vi "ADC Fetch From Digitizing Process.vi"(6 "stop ref":refnum<vi>, 8 "error in":errorcluster, 11 "adc session in":T3={"niScope"={"channel cfg"=[], "sessions"=[], "multi cards"=FALSE, "channels"=0, "type"=enum."n/a", "memory [B/chn]"=0, "ext. clock [Hz]"=0.0, "samples count"=0, "use streaming"=FALSE, "proc setup"={"packet size [smpl]"=0, "current timeout [s]"=0.0, "blk2blk timeout [s]"=0.0, "event time"=timestamp(0 s since 1904-01-01), "temp sampl T [s]"=0.0, "data queue"=refnum, "stop notifier"=refnum, "proc ref"=refnum}, "sample width [B]"=0, "ranges [V]"=[], "trigger setup"={"coupling"=1, "level [V]"=0.0, "slope"=0, "mode"=enum."Immediate"}, "fs [Hz]"=0.0, "bitres [bit]"=0}, "3458A"={"channels"=[], "sync unit"={"VISA"="", "type"=enum."Picotest U6200A"}, "awg unit"={"type"=enum."Agilent 331xxA to 332xxA", "VISA"="", "enable 10MHz ref"=FALSE}, "sync mode"=enum."MASTER-SLAVE, MASTER clocked by TIMER", "streaming mode"=FALSE, "idn mode"=enum."Auto", "sampling mode"=enum."DCV", "Ts [s]"=0.0, "sample memory [B]"=0, "proc setup"={"channel id"=0, "packet size [smpl]"=0, "current timeout [s]"=0.0, "blk2blk timeout [s]"=0.0, "event time"=timestamp(0 s since 1904-01-01), "stop notifier"=refnum, "data queues"=[], "proc refs"=[], "bus semaphore"=refnum}, "sample size [B]"=0, "sample count"=0, "aux data"={"channel id"=0, "valid?"=[], "gain [V]"=[], "timestamp [s]"=[], "Ts [s]"=0.0, "abs timestamp"=timestamp(0 s since 1904-01-01), "t [deg C]"=[]}, "ranges [V]"=[], "aperture [s]"=0.0, "LEVEL trigger"={"edge"=enum."POS", "level [V]"=0.0, "coupling"=enum."DC"}, "trigger mode"=enum."AUTO", "measure temp.?"=FALSE, "disp mesages"=[], "shared bus?"=FALSE, "disable display?"=FALSE, "aper mode"=enum."Manual", "aper rules"=[]}, "dsdll"={"dsdll"={"dsdll path"=path "", "dsdll handle"=[], "output devices"=[], "capture devices"=[]}, "channels"=0, "device id"=0, "channel idns"=[], "proc setup"={"packet size [smpl]"=0, "current timeout [s]"=0.0, "blk2blk timeout [s]"=0.0, "event time"=timestamp(0 s since 1904-01-01), "data queue"=refnum, "stop notifier"=refnum, "proc ref"=refnum}, "samples count"=0, "fs [Hz]"=0.0}, "type"=enum."niScope", "channel idn str"=[], "aux instr idn str"=[], "modified?"=FALSE, "simadc"={"channels"=[], "range [V]"=0.0, "Ts step [s]"=0.0, "time [s]"=0.0, "fs [Hz]"=0.0, "count"=0, "smpl offset"=0, "set count"=0, "bit res"=0}, "force rst?"=FALSE, "exit mode"=enum."Immediate reset", "exit dly"=0.0, "exit tmr"=timestamp(0 s since 1904-01-01), "busy?"=FALSE, "accessed?"=FALSE, "QuADC session"={"channel cfg"=[], "sessions"=[], "multi cards"=FALSE, "channels"=0, "type"=enum."n/a", "memory [B/chn]"=0, "ext. clock [Hz]"=0.0, "samples count"=0, "use streaming"=FALSE, "proc setup"={"packet size [smpl]"=0, "current timeout [s]"=0.0, "blk2blk timeout [s]"=0.0, "event time"=timestamp(0 s since 1904-01-01), "temp sampl T [s]"=0.0, "data queue"=refnum, "stop notifier"=refnum, "proc ref"=refnum}, "sample width [B]"=0, "ranges [V]"=[], "trigger setup"={"coupling"=1, "level [V]"=0.0, "slope"=0, "mode"=enum."Immediate"}, "fs [Hz]"=0.0, "bitres [bit]"=0}} {"QuADC session"."trigger setup"."level [V]" format="%.2f"; "QuADC session"."trigger setup"."coupling" items=["AC"=0, "DC"=1, "HF Reject"=3, "LF Reject"=4, "AC Plus HF Reject"=1001]; "QuADC session"."channel cfg"."Clock fr. (Hz)" min=0.0 format="%#_9p"; "QuADC session"."channel cfg"."Number of JJ" min=1; "QuADC session"."channel cfg"."Range [Vpk]" min=0.0; "QuADC session"."channel cfg"."Channel" min=0; "3458A"."channels"."Range [Vpk]" min=0.0; "niScope"."trigger setup"."level [V]" format="%.2f"; "niScope"."trigger setup"."coupling" items=["AC"=0, "DC"=1, "HF Reject"=3, "LF Reject"=4, "AC Plus HF Reject"=1001]; "niScope"."channel cfg"."Range [Vpk]" min=0.0; "niScope"."channel cfg"."Channel" min=0}) -> (0 "error out":errorcluster, 1 "aux data":T1, 2 "data packet":T2, 3 "adc session out":T3={"niScope"={"channel cfg"=[], "sessions"=[], "multi cards"=FALSE, "channels"=0, "type"=enum."n/a", "memory [B/chn]"=0, "ext. clock [Hz]"=0.0, "samples count"=0, "use streaming"=FALSE, "proc setup"={"packet size [smpl]"=0, "current timeout [s]"=0.0, "blk2blk timeout [s]"=0.0, "event time"=timestamp(0 s since 1904-01-01), "temp sampl T [s]"=0.0, "data queue"=refnum, "stop notifier"=refnum, "proc ref"=refnum}, "sample width [B]"=0, "ranges [V]"=[], "trigger setup"={"coupling"=1, "level [V]"=0.0, "slope"=0, "mode"=enum."Immediate"}, "fs [Hz]"=0.0, "bitres [bit]"=0}, "3458A"={"channels"=[], "sync unit"={"VISA"="", "type"=enum."Picotest U6200A"}, "awg unit"={"type"=enum."Agilent 331xxA to 332xxA", "VISA"="", "enable 10MHz ref"=FALSE}, "sync mode"=enum."MASTER-SLAVE, MASTER clocked by TIMER", "streaming mode"=FALSE, "idn mode"=enum."Auto", "sampling mode"=enum."DCV", "Ts [s]"=0.0, "sample memory [B]"=0, "proc setup"={"channel id"=0, "packet size [smpl]"=0, "current timeout [s]"=0.0, "blk2blk timeout [s]"=0.0, "event time"=timestamp(0 s since 1904-01-01), "stop notifier"=refnum, "data queues"=[], "proc refs"=[], "bus semaphore"=refnum}, "sample size [B]"=0, "sample count"=0, "aux data"={"channel id"=0, "valid?"=[], "gain [V]"=[], "timestamp [s]"=[], "Ts [s]"=0.0, "abs timestamp"=timestamp(0 s since 1904-01-01), "t [deg C]"=[]}, "ranges [V]"=[], "aperture [s]"=0.0, "LEVEL trigger"={"edge"=enum."POS", "level [V]"=0.0, "coupling"=enum."DC"}, "trigger mode"=enum."AUTO", "measure temp.?"=FALSE, "disp mesages"=[], "shared bus?"=FALSE, "disable display?"=FALSE, "aper mode"=enum."Manual", "aper rules"=[]}, "dsdll"={"dsdll"={"dsdll path"=path "", "dsdll handle"=[], "output devices"=[], "capture devices"=[]}, "channels"=0, "device id"=0, "channel idns"=[], "proc setup"={"packet size [smpl]"=0, "current timeout [s]"=0.0, "blk2blk timeout [s]"=0.0, "event time"=timestamp(0 s since 1904-01-01), "data queue"=refnum, "stop notifier"=refnum, "proc ref"=refnum}, "samples count"=0, "fs [Hz]"=0.0}, "type"=enum."niScope", "channel idn str"=[], "aux instr idn str"=[], "modified?"=FALSE, "simadc"={"channels"=[], "range [V]"=0.0, "Ts step [s]"=0.0, "time [s]"=0.0, "fs [Hz]"=0.0, "count"=0, "smpl offset"=0, "set count"=0, "bit res"=0}, "force rst?"=FALSE, "exit mode"=enum."Immediate reset", "exit dly"=0.0, "exit tmr"=timestamp(0 s since 1904-01-01), "busy?"=FALSE, "accessed?"=FALSE, "QuADC session"={"channel cfg"=[], "sessions"=[], "multi cards"=FALSE, "channels"=0, "type"=enum."n/a", "memory [B/chn]"=0, "ext. clock [Hz]"=0.0, "samples count"=0, "use streaming"=FALSE, "proc setup"={"packet size [smpl]"=0, "current timeout [s]"=0.0, "blk2blk timeout [s]"=0.0, "event time"=timestamp(0 s since 1904-01-01), "temp sampl T [s]"=0.0, "data queue"=refnum, "stop notifier"=refnum, "proc ref"=refnum}, "sample width [B]"=0, "ranges [V]"=[], "trigger setup"={"coupling"=1, "level [V]"=0.0, "slope"=0, "mode"=enum."Immediate"}, "fs [Hz]"=0.0, "bitres [bit]"=0}} {"QuADC session"."trigger setup"."level [V]" format="%.2f"; "QuADC session"."trigger setup"."coupling" items=["AC"=0, "DC"=1, "HF Reject"=3, "LF Reject"=4, "AC Plus HF Reject"=1001]; "QuADC session"."channel cfg"."Clock fr. (Hz)" min=0.0 format="%#_9p"; "QuADC session"."channel cfg"."Number of JJ" min=1; "QuADC session"."channel cfg"."Range [Vpk]" min=0.0; "QuADC session"."channel cfg"."Channel" min=0; "3458A"."channels"."Range [Vpk]" min=0.0; "niScope"."trigger setup"."level [V]" format="%.2f"; "niScope"."trigger setup"."coupling" items=["AC"=0, "DC"=1, "HF Reject"=3, "LF Reject"=4, "AC Plus HF Reject"=1001]; "niScope"."channel cfg"."Range [Vpk]" min=0.0; "niScope"."channel cfg"."Channel" min=0}, 4 "fetching done?":bool)   [LabVIEW 2018]
doc: "Call this in a loop to fetch sample data comming from running digitizing process(es). It fetches the sample data, merges them from particular channels to one array.\nIf some sample data are available or a status is updated it will be found in 'data packet' variable. Content of the variable is valid only if its flag 'valid?' is true. It contains data either in int32 or int16 format. Everytime some data are returned the 'count' of samples per channels is non-zero and 'offset' indicates relative position of first sample to the start of sampling. When digitizer is sampling (not just returning data) the flag 'sampling' is true. If supported by selected HW it will also return usage of intrument memory buffer and sample data queue. If not supported the value will be NaN. \nSecond output of the VI is 'aux data' which are returned only once per whole fetching sequence. It is valid if its flag 'valid?' is True. The aux. data contains 'gain' and 'offset' scaling factors needed to convert integer sample data to voltage. It will also return vector of measured temperatures and corresponding timestamps of measurement during the sampling if it is supported by the HW. Last parameter is a relative timestamp of first sample for each channel. \nCaller must check and process content of both 'data packet' and 'aux data' every time this VI is called. Fetching must be terminated when the function returnes error or returnes True on 'fetching done?' flag.\nVI modifies session content so do not assign just ADC session in!"
uses:
  ADC Session.ctl
  drivers/niScope/niScope Session.ctl
  drivers/niScope/niScope Virtual Channel Config.ctl
  drivers/niScope/niScope Virtual Channel Mode.ctl
  drivers/niScope/niScope Virtual Channel Input Z.ctl
  drivers/niScope/niScope Virtual Channel Coupling.ctl
  drivers/niScope/niScope Type.ctl
  drivers/niScope/niScope Digitizing Process Options.ctl
  drivers/niScope/niScope Data Packet.ctl
  drivers/niScope/niScope Trigger Setup.ctl
  <instrlib>/niScope/Controls/niScope trigger coupling.ctl
  <instrlib>/niScope/Controls/niScope trigger slope.ctl
  drivers/DMM/3458A Digitizer Session.ctl
  drivers/DMM/3458A Virtual Channel Config.ctl
  drivers/Counter/Counter Session.ctl
  drivers/Counter/Counter Type.ctl
  drivers/AWG/AWG Session.ctl
  drivers/AWG/AWG Type.ctl
  drivers/DMM/3458A Sync Mode.ctl
  drivers/DMM/3458A Idn Mode.ctl
  drivers/DMM/3458A Digitizing Low Levels/Configure/Sampling Mode.ctl
  drivers/DMM/3458A Digitizing Process Options.ctl
  drivers/DMM/3458A Data Packet.ctl
  drivers/DMM/3458A Aux Record Data.ctl
  drivers/DMM/3458A Digitizing Low Levels/Configure/Level Setup.ctl
  drivers/DMM/3458A Digitizing Low Levels/Configure/First Sample Trigger.ctl
  drivers/DMM/3458A Aperture Selection Mode.ctl
  drivers/dsdll/DSDLL Session.ctl
  drivers/dsdll/dsdll source distribution/dsdll_instance.ctl
  drivers/dsdll/dsdll source distribution/dsdll_device_record.ctl
  drivers/dsdll/DSDLL Process Config.ctl
  drivers/dsdll/DSDLL Data Packet.ctl
  ADC Type.ctl
  drivers/simulated_adc/SimAdc Config.ctl
  drivers/simulated_adc/SimAdc Channel Cfg.ctl
  ADC On Close Action.ctl
  drivers/Quatsch_driver/QuADCDriver/QuADC Session.ctl
  drivers/Quatsch_driver/QuADCDriver/QuADC Virtual Channel Config.ctl
  drivers/Quatsch_driver/QuADCDriver/QuADC Virtual Channel Mode.ctl
  drivers/Quatsch_driver/QuADCDriver/QuADC Virtual Channel Input Z.ctl
  drivers/Quatsch_driver/QuADCDriver/QuADC Virtual Channel Coupling.ctl
  drivers/Quatsch_driver/QuADCDriver/QuADC Type.ctl
  drivers/Quatsch_driver/QuADCDriver/QuADC Digitizing Process Options.ctl
  drivers/Quatsch_driver/QuADCDriver/QuADC Data Packet.ctl
  drivers/Quatsch_driver/QuADCDriver/QuADC Trigger Setup.ctl
  ADC Data Packet.ctl
  ADC Aux Data.ctl
  drivers/niScope/niScope Virtual Digitizer.lvlib
  drivers/DMM/3458A Virtual Digitizer.lvlib
  drivers/dsdll/DSDLL Virtual Digitizer.lvlib
  <vilib>/Utility/error.llb/Error Cluster From Error Code.vi
  <vilib>/ErrorRing/Error Ring.xnode
  drivers/Quatsch_driver/QuADCDriver/QuADC Virtual Digitizer.lvlib
  drivers/Counter/Counter.lvlib
  drivers/AWG/AWG.lvlib
  drivers/DMM/3458A Digitizing Low Levels/3458A Digitizing Low Levels.lvlib
  drivers/dsdll/dsdll source distribution/dsdll.lvlib
panel:
  # "IP Address"
  # "."
  # "."
  # "."
  # ":"
  # "IP Address"
  # "."
  # "."
  # "."
  # ":"
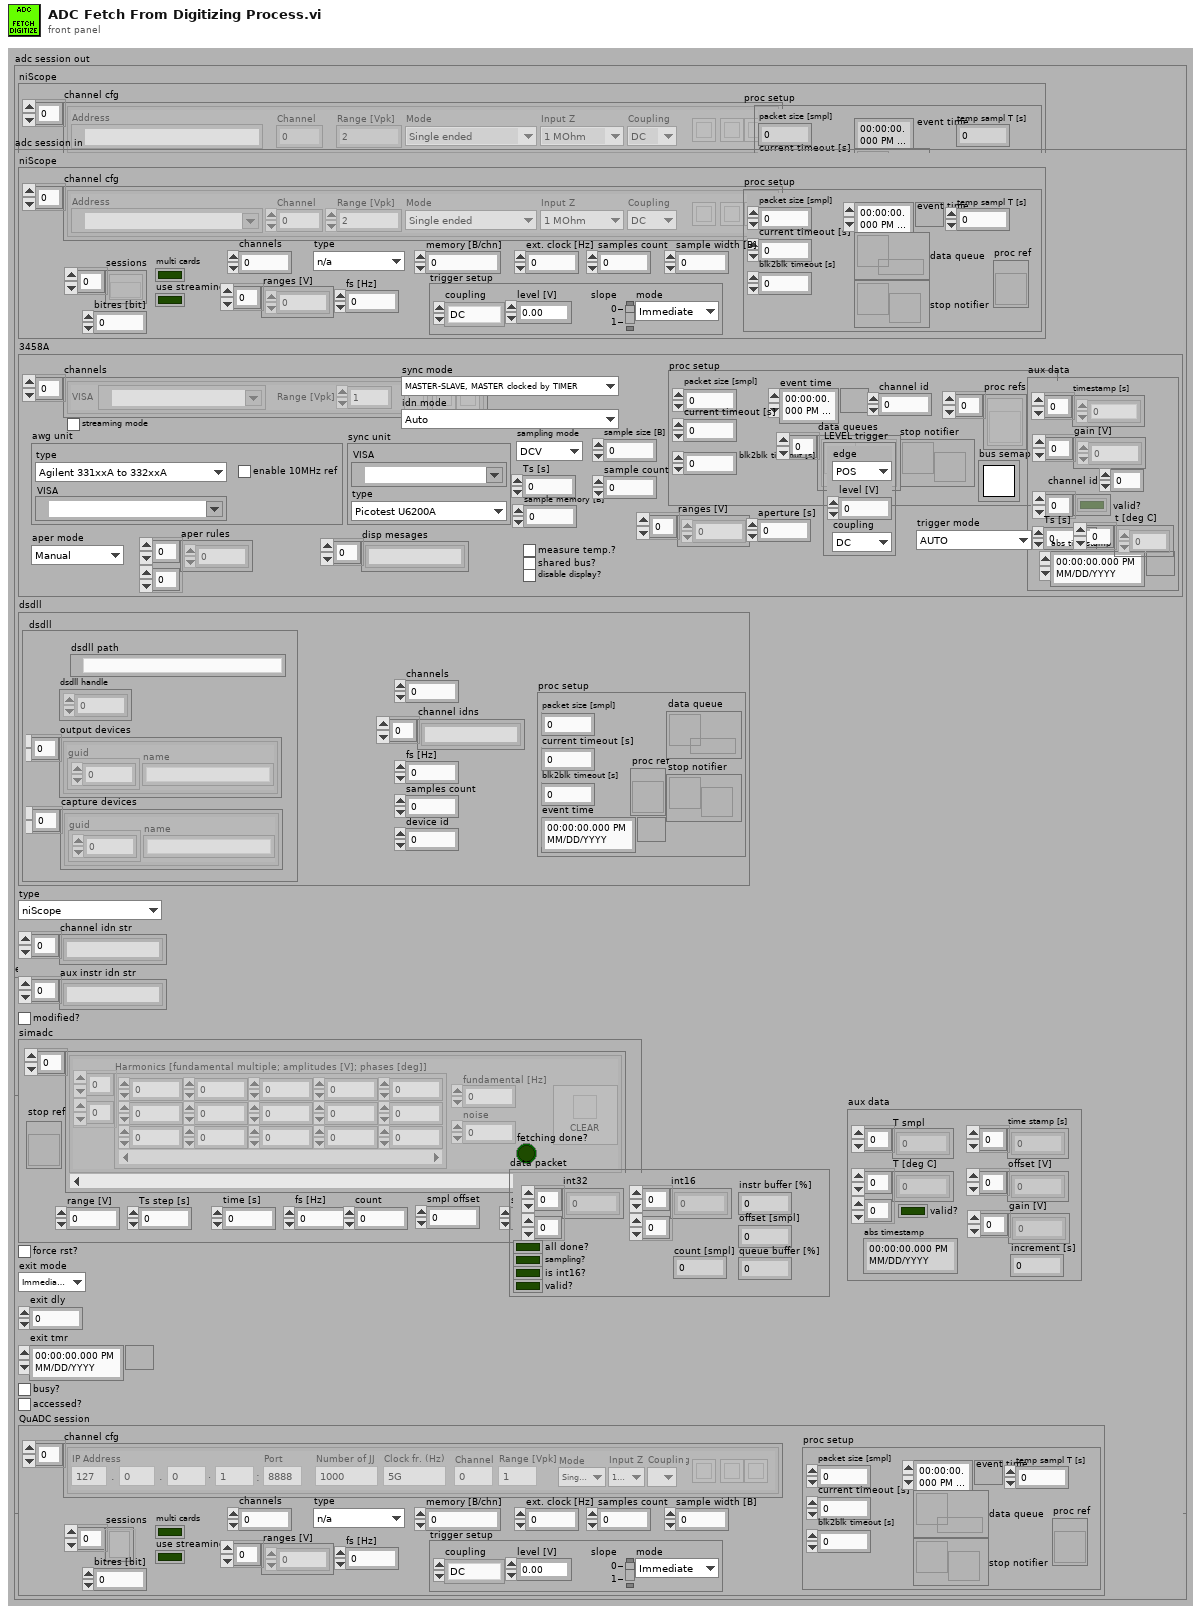
[diagram p1: front panel]
types:
  T1 = typedef "ADC Aux Data.ctl" = cluster{"offset [V]":dbl[], "gain [V]":dbl[], "time stamp [s]":dbl[], "increment [s]":dbl, "T smpl":i64[], "T [deg C]":dbl[][], "valid?":bool, "abs timestamp":timestamp}
  T2 = typedef "ADC Data Packet.ctl" = cluster{"int32":i32[][], "int16":i16[][], "offset [smpl]":i64, "count [smpl]":i32, "is int16?":bool, "all done?":bool, "sampling?":bool, "instr buffer [%]":dbl, "queue buffer [%]":dbl, "valid?":bool}
  T3 = typedef "ADC Session.ctl" = cluster{"niScope":T4, "3458A":T14, "dsdll":T29, "type":T33, "channel idn str":string[], "aux instr idn str":string[], "modified?":bool, "simadc":T34, "force rst?":bool, "exit mode":T36, "exit dly":dbl, "exit tmr":timestamp, "busy?":bool, "accessed?":bool, "QuADC session":T37}
  T4 = typedef "niScope Virtual Digitizer.lvlib/niScope Session.ctl" = cluster{"channel cfg":T5[], "sessions":refnum<k20>[], "multi cards":bool, "channels":i32, "type":T9, "memory [B/chn]":i32, "ext. clock [Hz]":dbl, "samples count":i64, "use streaming":bool, "proc setup":T10, "sample width [B]":i32, "ranges [V]":dbl[], "trigger setup":T11, "fs [Hz]":dbl, "bitres [bit]":i32}
  T5 = typedef "niScope Virtual Digitizer.lvlib/niScope Virtual Channel Config.ctl" = cluster{"Address":refnum<k15>, "Channel":i32, "Mode":T6, "Input Z":T7, "Coupling":T8, "Range [Vpk]":dbl, "btn clr":bool, "btn up":bool, "btn down":bool}
  T6 = typedef "niScope Virtual Digitizer.lvlib/niScope Virtual Channel Mode.ctl" = enum16{"Single ended", "Unbal. differential", "Differential"}
  T7 = typedef "niScope Virtual Digitizer.lvlib/niScope Virtual Channel Input Z.ctl" = enum16{"1 MOhm", "50 Ohm"}
  T8 = typedef "niScope Virtual Digitizer.lvlib/niScope Virtual Channel Coupling.ctl" = enum16{"AC", "DC", "GND"}
  T9 = typedef "niScope Virtual Digitizer.lvlib/niScope Type.ctl" = enum16{"n/a", "5922"}
  T10 = typedef "niScope Virtual Digitizer.lvlib/niScope Digitizing Process Options.ctl" = cluster{"packet size [smpl]":i64, "current timeout [s]":dbl, "blk2blk timeout [s]":dbl, "event time":timestamp, "temp sampl T [s]":dbl, "data queue":refnum<queue>, "stop notifier":refnum<notifier>, "proc ref":refnum<vi>}
  T11 = typedef "niScope Virtual Digitizer.lvlib/niScope Trigger Setup.ctl" = cluster{"coupling":T12, "level [V]":dbl, "slope":T13, "mode":enum16{"Immediate", "External", "Level"}}
  T12 = typedef "niScope trigger coupling.ctl" = u16
  T13 = typedef "niScope trigger slope.ctl" = i32
  T14 = typedef "3458A Virtual Digitizer.lvlib/3458A Digitizer Session.ctl" = cluster{"channels":T15[], "sync unit":T16, "awg unit":T18, "sync mode":T20, "streaming mode":bool, "idn mode":T21, "sampling mode":T22, "Ts [s]":dbl, "sample memory [B]":i32, "proc setup":T23, "sample size [B]":i32, "sample count":i32, "aux data":T25, "ranges [V]":dbl[], "aperture [s]":dbl, "LEVEL trigger":T26, "trigger mode":T27, "measure temp.?":bool, "disp mesages":string[], "shared bus?":bool, "disable display?":bool, "aper mode":T28, "aper rules":dbl[][]}
  T15 = typedef "3458A Virtual Digitizer.lvlib/3458A Virtual Channel Config.ctl" = cluster{"VISA":refnum<visa-resource-name>, "Range [Vpk]":dbl, "btn clr":bool, "btn up":bool, "btn down":bool}
  T16 = typedef "Counter.lvlib/Counter Session.ctl" = cluster{"VISA":refnum<visa-resource-name>, "type":T17}
  T17 = typedef "Counter.lvlib/Counter Type.ctl" = enum16{"Picotest U6200A", "dummy"}
  T18 = typedef "AWG.lvlib/AWG Session.ctl" = cluster{"type":T19, "VISA":refnum<visa-resource-name>, "enable 10MHz ref":bool}
  T19 = typedef "AWG.lvlib/AWG Type.ctl" = enum16{"Agilent 331xxA to 332xxA", "Agilent 335xxA to 336xxA", "Tektronix AFG3101C", "dummy"}
  T20 = typedef "3458A Virtual Digitizer.lvlib/3458A Sync Mode.ctl" = enum16{"MASTER-SLAVE, MASTER clocked by TIMER", "MASTER-SLAVE, MASTER clocked by AWG", "ALL clocked by AWG", "MASTER-SLAVE, ALL clocked by TIMER", "ALL clocked by AWG with DFLL"}
  T21 = typedef "3458A Virtual Digitizer.lvlib/3458A Idn Mode.ctl" = enum16{"Auto", "Sequential (chn A, chn B, ...)", "From calibration string"}
  T22 = typedef "3458A Virtual Digitizer.lvlib/3458A Digitizing Low Levels.lvlib/Sampling Mode.ctl" = enum16{"DCV", "DSDC", "DSAC"}
  T23 = typedef "3458A Virtual Digitizer.lvlib/3458A Digitizing Process Options.ctl" = cluster{"channel id":i32, "packet size [smpl]":i32, "current timeout [s]":dbl, "blk2blk timeout [s]":dbl, "event time":timestamp, "stop notifier":refnum<notifier>, "data queues":refnum<queue>[], "proc refs":refnum<vi>[], "bus semaphore":T24}
  T24 = typedef "Semaphore RefNum" = refnum<k1>
  T25 = typedef "3458A Virtual Digitizer.lvlib/3458A Aux Record Data.ctl" = cluster{"channel id":i32, "valid?":bool[], "gain [V]":dbl[], "timestamp [s]":dbl[], "Ts [s]":dbl, "abs timestamp":timestamp, "t [deg C]":dbl[]}
  T26 = typedef "3458A Virtual Digitizer.lvlib/3458A Digitizing Low Levels.lvlib/Level Setup.ctl" = cluster{"edge":enum16{"POS", "NEG"}, "level [V]":dbl, "coupling":enum16{"DC", "AC"}}
  T27 = typedef "3458A Virtual Digitizer.lvlib/3458A Digitizing Low Levels.lvlib/First Sample Trigger.ctl" = enum16{"AUTO", "EXT", "SYN", "SGL", "HOLD", "LEVEL"}
  T28 = typedef "3458A Virtual Digitizer.lvlib/3458A Aperture Selection Mode.ctl" = enum16{"Manual", "Maximum", "Table"}
  T29 = typedef "DSDLL Virtual Digitizer.lvlib/DSDLL Session.ctl" = cluster{"dsdll":T30, "channels":i32, "device id":i32, "channel idns":string[], "proc setup":T32, "samples count":i32, "fs [Hz]":dbl}
  T30 = typedef "dsdll.lvlib/dsdll_instance.ctl" = cluster{"dsdll path":path, "dsdll handle":u8[], "output devices":T31[], "capture devices":T31[]}
  T31 = typedef "dsdll.lvlib/dsdll_device_record.ctl" = cluster{"guid":u8[], "name":string}
  T32 = typedef "DSDLL Virtual Digitizer.lvlib/DSDLL Process Config.ctl" = cluster{"packet size [smpl]":i32, "current timeout [s]":dbl, "blk2blk timeout [s]":dbl, "event time":timestamp, "data queue":refnum<queue>, "stop notifier":refnum<notifier>, "proc ref":refnum<vi>}
  T33 = typedef "ADC Type.ctl" = enum16{"niScope", "3458A", "DirectSound DLL", "dummy", "QuADC"}
  T34 = typedef "SimAdc Config.ctl" = cluster{"channels":T35[], "range [V]":dbl, "Ts step [s]":dbl, "time [s]":dbl, "fs [Hz]":dbl, "count":i64, "smpl offset":i64, "set count":i64, "bit res":i32}
  T35 = typedef "SimAdc Channel Cfg.ctl" = cluster{"harmonics":dbl[][], "btn clear":bool, "noise":dbl, "fundamental [Hz]":dbl}
  T36 = typedef "ADC On Close Action.ctl" = enum16{"Immediate reset", "Delayed reset"}
  T37 = typedef "QuADC Virtual Digitizer.lvlib/QuADC Session.ctl" = cluster{"channel cfg":T38[], "sessions":refnum<k5>[], "multi cards":bool, "channels":i32, "type":T42, "memory [B/chn]":i32, "ext. clock [Hz]":dbl, "samples count":i64, "use streaming":bool, "proc setup":T43, "sample width [B]":i32, "ranges [V]":dbl[], "trigger setup":T44, "fs [Hz]":dbl, "bitres [bit]":i32}
  T38 = typedef "QuADC Virtual Digitizer.lvlib/QuADC Virtual Channel Config.ctl" = cluster{"Channel":i32, "Mode":T39, "Input Z":T40, "Coupling":T41, "Range [Vpk]":dbl, "btn clr":bool, "btn up":bool, "btn down":bool, "IP address A":u8, "IP address B":u8, "IP address C":u8, "IP address D":u8, "Port":u16, "Number of JJ":u32, "Clock fr. (Hz)":dbl}
  T39 = typedef "QuADC Virtual Digitizer.lvlib/QuADC Virtual Channel Mode.ctl" = enum16{"Single ended", "Unbal. differential", "Differential"}
  T40 = typedef "QuADC Virtual Digitizer.lvlib/QuADC Virtual Channel Input Z.ctl" = enum16{"1 MOhm", "50 Ohm"}
  T41 = typedef "QuADC Virtual Digitizer.lvlib/QuADC Virtual Channel Coupling.ctl" = enum16{"AC", "DC", "GND"}
  T42 = typedef "QuADC Virtual Digitizer.lvlib/QuADC Type.ctl" = enum16{"n/a", "v1"}
  T43 = typedef "QuADC Virtual Digitizer.lvlib/QuADC Digitizing Process Options.ctl" = cluster{"packet size [smpl]":i64, "current timeout [s]":dbl, "blk2blk timeout [s]":dbl, "event time":timestamp, "temp sampl T [s]":dbl, "data queue":refnum<queue>, "stop notifier":refnum<notifier>, "proc ref":refnum<vi>}
  T44 = typedef "QuADC Virtual Digitizer.lvlib/QuADC Trigger Setup.ctl" = cluster{"coupling":T12, "level [V]":dbl, "slope":T13, "mode":enum16{"Immediate", "External", "Level"}}
  T45 = typedef "niScope Virtual Digitizer.lvlib/niScope Record Aux Data.ctl" = cluster{"T smpl":i64[], "T [deg C]":dbl[][], "time stamp [s]":dbl[], "offset":dbl[], "gain":dbl[], "increment [s]":dbl, "valid?":bool, "abs timestamp":timestamp}
  T46 = typedef "niScope Virtual Digitizer.lvlib/niScope Data Packet.ctl" = cluster{"int32":i32[][], "card buffer [%]":dbl, "all done?":bool, "offset [smpl]":i64, "sampling?":bool, "queue buffer [%]":dbl, "int16":i16[][], "is int16?":bool, "count [smpl]":i32, "valid?":bool}
  T47 = typedef "QuADC Virtual Digitizer.lvlib/QuADC Record Aux Data.ctl" = cluster{"T smpl":i64[], "T [deg C]":dbl[][], "time stamp [s]":dbl[], "offset":dbl[], "gain":dbl[], "increment [s]":dbl, "valid?":bool, "abs timestamp":timestamp}
  T48 = typedef "QuADC Virtual Digitizer.lvlib/QuADC Data Packet.ctl" = cluster{"int32":i32[][], "card buffer [%]":dbl, "all done?":bool, "offset [smpl]":i64, "sampling?":bool, "queue buffer [%]":dbl, "int16":i16[][], "is int16?":bool, "count [smpl]":i32, "valid?":bool}
  T49 = typedef "3458A Virtual Digitizer.lvlib/3458A Data Packet.ctl" = cluster{"data":i32[][], "offset [smpl]":i32, "count [smpl]":i32, "all done?":bool, "sampling?":bool, "queue buffer [%]":dbl, "valid?":bool}
  T50 = typedef "DSDLL Virtual Digitizer.lvlib/DSDLL Aux Record Data.ctl" = cluster{"time stamp [s]":dbl[], "gain":dbl[], "increment [s]":dbl, "valid?":bool, "abs timestamp":timestamp}
  T51 = typedef "DSDLL Virtual Digitizer.lvlib/DSDLL Data Packet.ctl" = cluster{"int32":i32[][], "card buffer [%]":dbl, "all done?":bool, "offset [smpl]":i32, "sampling?":bool, "queue buffer [%]":dbl, "count [smpl]":i32, "valid?":bool}
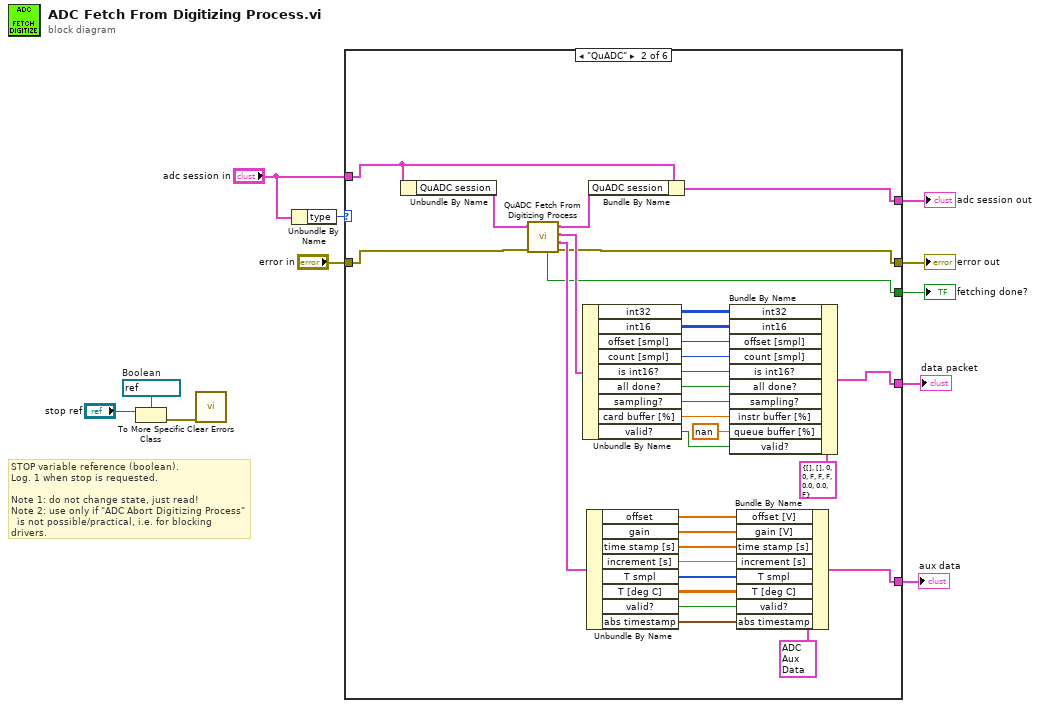
[diagram p0: block diagram]
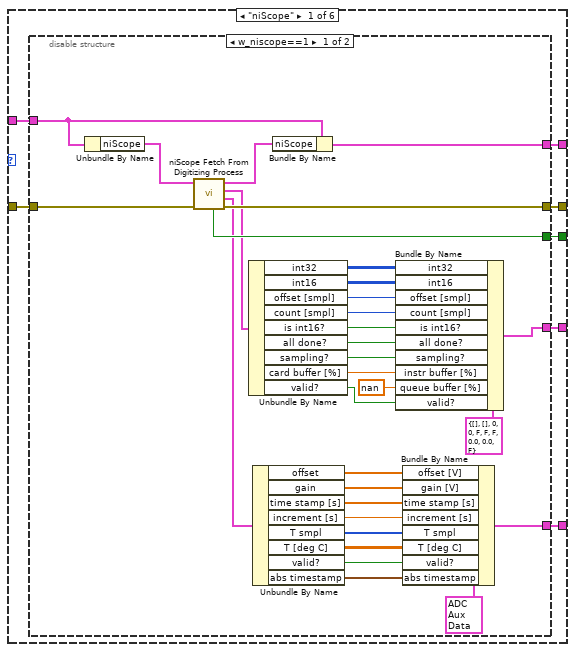
[diagram p2: hidden frame]
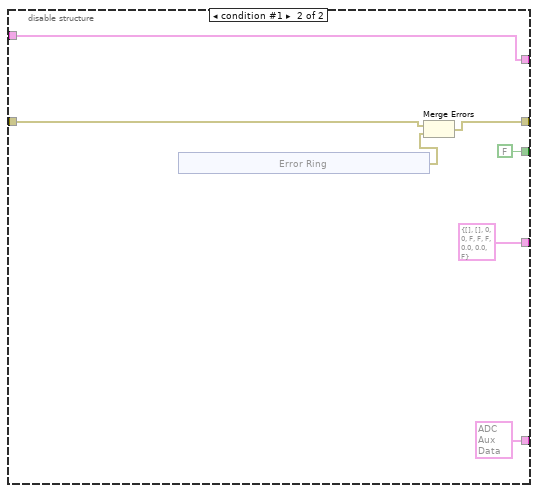
[diagram p3: hidden frame]
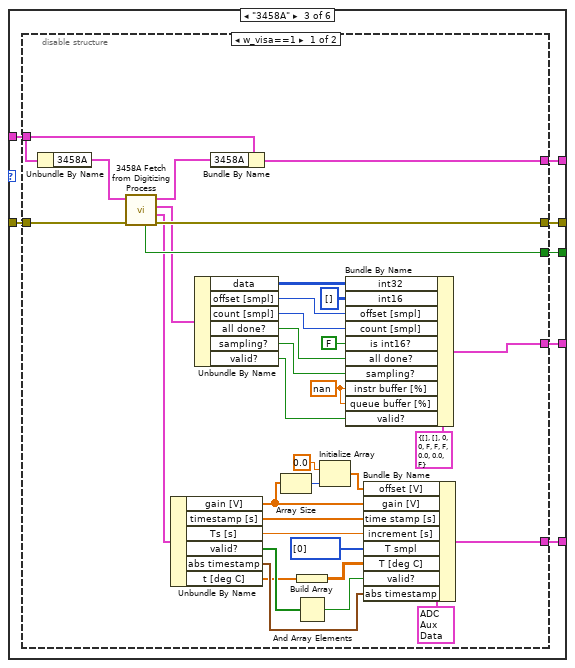
[diagram p4: hidden frame]
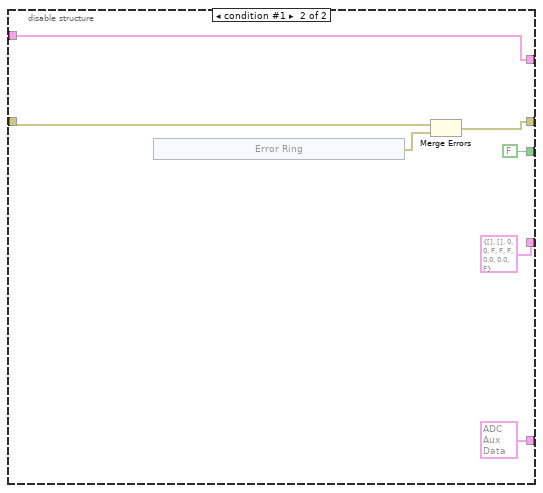
[diagram p5: hidden frame]
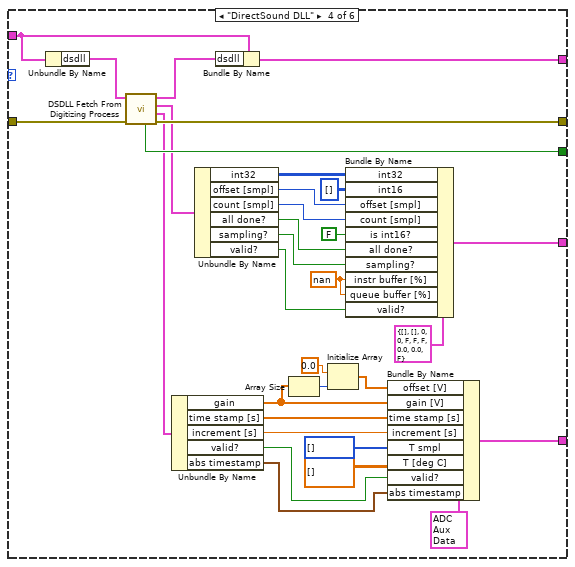
[diagram p6: hidden frame]
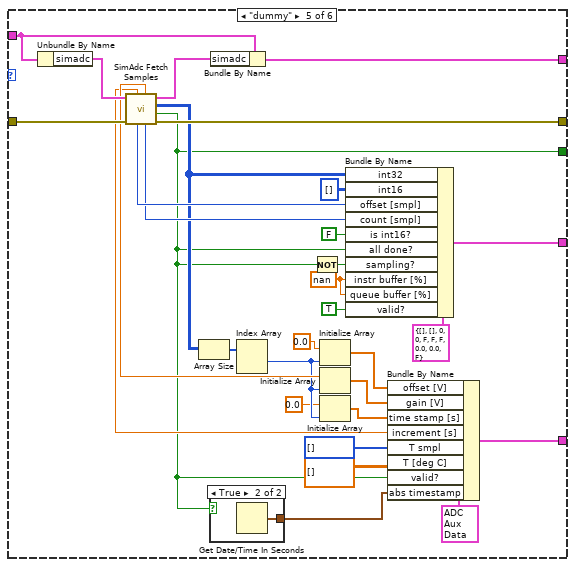
[diagram p7: hidden frame]
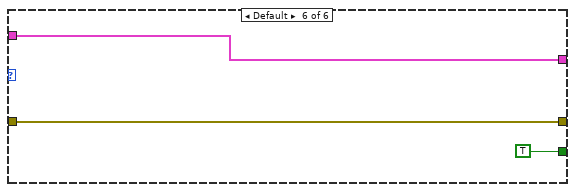
[diagram p9: hidden frame]
diagram:
  w1 = refnum<vi> refnum  # Boolean
  # "STOP variable reference (boolean).\nLog. 1 when stop is requested.\n\nNote 1: do not change state, just read!\nNote 2: use only if \"ADC Abort Digitizing Process\"\n  is not possible/practical, i.e. for blocking drivers."
  n1 = To More Specific Class(target class=w1, reference="stop ref") -> (error out=w2:errorcluster)  [unwired: 1 in, 1 out]
  n2 = call <vilib>:"Clear Errors.vi"("error in (no error)"=w2) -> ()  [unwired: 5 in, 2 out]
  n3 = Unbundle By Name("adc session in") -> ("type"=w11:T33)
  n4 = case shown="\"QuADC\"" w11 {
    tunnel: "error in" -> [w18 w63 w99 w177 w208 w212]
    tunnel: "adc session in" -> [w17 w92 w98 w175 w206 w211]
    tunnel: [w16 w91 w97 w174 w205 w211] -> w8
    tunnel: [w15 w64 w96 w173 w204 w212] -> w7
    tunnel: [w14 w62 w95 w172 w179 TRUE] -> w6
    tunnel: [w13 w90 w94 w170 w202 _] -> w5
    tunnel: [w12 w89 w93 w159 w197 _] -> w4
    frame "niScope" {
      n5 = disable-structure shown="w_niscope==1" {
        disable-tunnel: w18 -> [w49 w55]
        disable-tunnel: w17 -> [w47 w53]
        disable-tunnel: [w45 w53] -> w16
        disable-tunnel: [w44 w54] -> w15
        disable-tunnel: [w43 FALSE ("fetching done?")] -> w14
        disable-tunnel: [w30 T2 {"int32"=[], "int16"=[], "offset [smpl]"=0, "count [smpl]"=0, "is int16?"=FALSE, "all done?"=FALSE, "sampling?"=FALSE, "instr buffer [%]"=0.0, "queue buffer [%]"=0.0, "valid?"=FALSE} ("data")] -> w13
        disable-tunnel: [w20 T1 {"offset [V]"=[], "gain [V]"=[], "time stamp [s]"=[], "increment [s]"=0.0, "T smpl"=[], "T [deg C]"=[], "valid?"=FALSE, "abs timestamp"=timestamp(0 s since 1904-01-01)} ("aux data")] -> w12
        frame condition #0 (active) {
          n6 = Unbundle By Name(w47) -> ("niScope"=w48:T4)
          n7 = call "niScope Fetch From Digitizing Process.vi"("error in"=w49, "niScope in"=w48) -> ("error out"=w44:errorcluster, "auxiliary sampling data"=w29:T45, "data block"=w41:T46, "niScope out"=w46:T4, "fetching done?"=w43:bool)  [unwired: 5 in]
          n8 = Unbundle By Name(w41) -> ("int32"=w40:i32[][], "int16"=w39:i16[][], "offset [smpl]"=w38:i64, "count [smpl]"=w37:i32, "is int16?"=w36:bool, "all done?"=w35:bool, "sampling?"=w34:bool, "card buffer [%]"=w33:dbl, "valid?"=w31:bool)
          n9 = Unbundle By Name(w29) -> ("offset"=w27:dbl[], "gain"=w26:dbl[], "time stamp [s]"=w25:dbl[], "increment [s]"=w24:dbl, "T smpl"=w23:i64[], "T [deg C]"=w22:dbl[][], "valid?"=w21:bool, "abs timestamp"=w19:timestamp)
          n10 = Bundle By Name(cluster=w47, "niScope"=w46) -> (w45:T3)
          n11 = Bundle By Name(cluster=T2 {"int32"=[], "int16"=[], "offset [smpl]"=0, "count [smpl]"=0, "is int16?"=FALSE, "all done?"=FALSE, "sampling?"=FALSE, "instr buffer [%]"=0.0, "queue buffer [%]"=0.0, "valid?"=FALSE} ("data"), "int32"=w40, "int16"=w39, "offset [smpl]"=w38, "count [smpl]"=w37, "is int16?"=w36, "all done?"=w35, "sampling?"=w34, "instr buffer [%]"=w33, "queue buffer [%]"=nan, "valid?"=w31) -> (w30:T2)
          n12 = Bundle By Name(cluster=T1 {"offset [V]"=[], "gain [V]"=[], "time stamp [s]"=[], "increment [s]"=0.0, "T smpl"=[], "T [deg C]"=[], "valid?"=FALSE, "abs timestamp"=timestamp(0 s since 1904-01-01)} ("aux data"), "offset [V]"=w27, "gain [V]"=w26, "time stamp [s]"=w25, "increment [s]"=w24, "T smpl"=w23, "T [deg C]"=w22, "valid?"=w21, "abs timestamp"=w19) -> (w20:T1)
        }
        frame condition #1 {
          n13 = xnode "Error Ring"() -> ("error out"=w56:errorcluster)
          n14 = Merge Errors(w55, w56) -> (w54:errorcluster)
        }
      }
    }
    frame "QuADC" {
      n15 = Unbundle By Name(w92) -> ("QuADC session"=w68:T37)
      n16 = call "QuADC Fetch From Digitizing Process.vi"("error in"=w63, "QuADC in"=w68) -> ("error out"=w64:errorcluster, "auxiliary sampling data"=w65:T47, "data block"=w66:T48, "QuADC out"=w67:T37, "fetching done?"=w62:bool)  [unwired: 5 in]
      n17 = Unbundle By Name(w66) -> ("int32"=w87:i32[][], "int16"=w86:i16[][], "offset [smpl]"=w85:i64, "count [smpl]"=w84:i32, "is int16?"=w83:bool, "all done?"=w82:bool, "sampling?"=w81:bool, "card buffer [%]"=w80:dbl, "valid?"=w78:bool)
      n18 = Unbundle By Name(w65) -> ("offset"=w76:dbl[], "gain"=w75:dbl[], "time stamp [s]"=w74:dbl[], "increment [s]"=w73:dbl, "T smpl"=w72:i64[], "T [deg C]"=w71:dbl[][], "valid?"=w70:bool, "abs timestamp"=w69:timestamp)
      n19 = Bundle By Name(cluster=w92, "QuADC session"=w67) -> (w91:T3)
      n20 = Bundle By Name(cluster=T2 {"int32"=[], "int16"=[], "offset [smpl]"=0, "count [smpl]"=0, "is int16?"=FALSE, "all done?"=FALSE, "sampling?"=FALSE, "instr buffer [%]"=0.0, "queue buffer [%]"=0.0, "valid?"=FALSE} ("data"), "int32"=w87, "int16"=w86, "offset [smpl]"=w85, "count [smpl]"=w84, "is int16?"=w83, "all done?"=w82, "sampling?"=w81, "instr buffer [%]"=w80, "queue buffer [%]"=nan, "valid?"=w78) -> (w90:T2)
      n21 = Bundle By Name(cluster=T1 {"offset [V]"=[], "gain [V]"=[], "time stamp [s]"=[], "increment [s]"=0.0, "T smpl"=[], "T [deg C]"=[], "valid?"=FALSE, "abs timestamp"=timestamp(0 s since 1904-01-01)} ("aux data"), "offset [V]"=w76, "gain [V]"=w75, "time stamp [s]"=w74, "increment [s]"=w73, "T smpl"=w72, "T [deg C]"=w71, "valid?"=w70, "abs timestamp"=w69) -> (w89:T1)
    }
    frame "3458A" {
      n22 = disable-structure shown="w_visa==1" {
        disable-tunnel: w99 -> [w133 w139]
        disable-tunnel: w98 -> [w131 w134]
        disable-tunnel: [w130 w134] -> w97
        disable-tunnel: [w129 w138] -> w96
        disable-tunnel: [w127 FALSE ("fetching done?")] -> w95
        disable-tunnel: [w125 T2 {"int32"=[], "int16"=[], "offset [smpl]"=0, "count [smpl]"=0, "is int16?"=FALSE, "all done?"=FALSE, "sampling?"=FALSE, "instr buffer [%]"=0.0, "queue buffer [%]"=0.0, "valid?"=FALSE} ("data")] -> w94
        disable-tunnel: [w112 T1 {"offset [V]"=[], "gain [V]"=[], "time stamp [s]"=[], "increment [s]"=0.0, "T smpl"=[], "T [deg C]"=[], "valid?"=FALSE, "abs timestamp"=timestamp(0 s since 1904-01-01)} ("aux data")] -> w93
        frame condition #0 (active) {
          w116 = nan ("instr buffer [%]")
          n23 = Unbundle By Name(w131) -> ("3458A"=w128:T14)
          n24 = call "3458A Fetch from Digitizing Process.vi"("error in"=w133, "session in"=w128) -> ("error out"=w129:errorcluster, "aux data"=w114:T25, "data packet"=w124:T49, "session out"=w132:T14, "fetching done?"=w127:bool)  [unwired: 5 in]
          n25 = Unbundle By Name(w114) -> ("gain [V]"=w106:dbl[], "timestamp [s]"=w111:dbl[], "Ts [s]"=w110:dbl, "valid?"=w108:bool[], "abs timestamp"=w102:timestamp, "t [deg C]"=w101:dbl[])
          n26 = Unbundle By Name(w124) -> ("data"=w121:i32[][], "offset [smpl]"=w122:i32, "count [smpl]"=w117:i32, "all done?"=w119:bool, "sampling?"=w118:bool, "valid?"=w115:bool)
          n27 = Bundle By Name(cluster=w131, "3458A"=w132) -> (w130:T3)
          n28 = Array Size(array=w106) -> (size(s)=w105:i32)
          n29 = Build Array(w101) -> (w100:dbl[][])
          n30 = And Array Elements(Boolean array=w108) -> (logical AND=w107:bool)
          n31 = Initialize Array(0.0 ("offset"), w105) -> (w104:dbl[])
          n32 = Bundle By Name(cluster=T2 {"int32"=[], "int16"=[], "offset [smpl]"=0, "count [smpl]"=0, "is int16?"=FALSE, "all done?"=FALSE, "sampling?"=FALSE, "instr buffer [%]"=0.0, "queue buffer [%]"=0.0, "valid?"=FALSE} ("data"), "int32"=w121, "int16"=i16[][] [], "offset [smpl]"=w122, "count [smpl]"=w117, "is int16?"=FALSE, "all done?"=w119, "sampling?"=w118, "instr buffer [%]"=w116, "queue buffer [%]"=w116, "valid?"=w115) -> (w125:T2)
          n33 = Bundle By Name(cluster=T1 {"offset [V]"=[], "gain [V]"=[], "time stamp [s]"=[], "increment [s]"=0.0, "T smpl"=[], "T [deg C]"=[], "valid?"=FALSE, "abs timestamp"=timestamp(0 s since 1904-01-01)} ("aux data"), "offset [V]"=w104, "gain [V]"=w106, "time stamp [s]"=w111, "increment [s]"=w110, "T smpl"=i32[] [0], "T [deg C]"=w100, "valid?"=w107, "abs timestamp"=w102) -> (w112:T1)
        }
        frame condition #1 {
          n34 = xnode "Error Ring"() -> ("error out"=w140:errorcluster)
          n35 = Merge Errors(w139, w140) -> (w138:errorcluster)
        }
      }
    }
    frame "DirectSound DLL" {
      w162 = nan ("instr buffer [%]")
      n36 = Unbundle By Name(w175) -> ("dsdll"=w152:T29)
      n37 = call "DSDLL Fetch From Digitizing Process.vi"("error in"=w177, "dsdll in"=w152) -> ("error out"=w173:errorcluster, "auxiliary sampling data"=w154:T50, "data block"=w153:T51, "dsdll out"=w176:T29, "fetching done?"=w172:bool)  [unwired: 5 in]
      n38 = Unbundle By Name(w154) -> ("gain"=w148:dbl[], "time stamp [s]"=w158:dbl[], "increment [s]"=w157:dbl, "valid?"=w151:bool, "abs timestamp"=w146:timestamp)
      n39 = Unbundle By Name(w153) -> ("int32"=w167:i32[][], "offset [smpl]"=w168:i32, "count [smpl]"=w163:i32, "all done?"=w165:bool, "sampling?"=w164:bool, "valid?"=w161:bool)
      n40 = Bundle By Name(cluster=w175, "dsdll"=w176) -> (w174:T3)
      n41 = Array Size(array=w148) -> (size(s)=w150:i32)
      n42 = Initialize Array(0.0 ("offset"), w150) -> (w147:dbl[])
      n43 = Bundle By Name(cluster=T2 {"int32"=[], "int16"=[], "offset [smpl]"=0, "count [smpl]"=0, "is int16?"=FALSE, "all done?"=FALSE, "sampling?"=FALSE, "instr buffer [%]"=0.0, "queue buffer [%]"=0.0, "valid?"=FALSE} ("data"), "int32"=w167, "int16"=i16[][] [], "offset [smpl]"=w168, "count [smpl]"=w163, "is int16?"=FALSE, "all done?"=w165, "sampling?"=w164, "instr buffer [%]"=w162, "queue buffer [%]"=w162, "valid?"=w161) -> (w170:T2)
      n44 = Bundle By Name(cluster=T1 {"offset [V]"=[], "gain [V]"=[], "time stamp [s]"=[], "increment [s]"=0.0, "T smpl"=[], "T [deg C]"=[], "valid?"=FALSE, "abs timestamp"=timestamp(0 s since 1904-01-01)} ("aux data"), "offset [V]"=w147, "gain [V]"=w148, "time stamp [s]"=w158, "increment [s]"=w157, "T smpl"=i32[] [], "T [deg C]"=dbl[][] [], "valid?"=w151, "abs timestamp"=w146) -> (w159:T1)
    }
    frame "dummy" {
      w199 = nan ("instr buffer [%]")
      n45 = Unbundle By Name(w206) -> ("simadc"=w188:T34)
      n46 = call "SimAdc Fetch Samples.vi"("error in"=w208, "simadc in"=w188) -> ("error out"=w204:errorcluster, "done"=w179:bool, "sample data"=w187:i32[][], "simadc out"=w207:T34, "samples fetched"=w191:i64, "scale factor [V]"=w185:dbl, "smpl offset"=w192:i64, "Ts [s]"=w180:dbl)  [unwired: 2 in]
      n47 = Array Size(array=w187) -> (size(s)=w186:i32[])
      n48 = case shown="True" w179 {
        tunnel: [_ w209] -> w178
        frame False {
        }
        frame True {
          n49 = Get Date/Time In Seconds() -> (seconds since 1Jan1904=w209:timestamp)
        }
      }
      n50 = Bundle By Name(cluster=w206, "simadc"=w207) -> (w205:T3)
      n51 = Index Array(array=w186) -> (element #1=w182:i32)  [unwired: 2 in, 1 out]
      n52 = Not(x=w179) -> (.not. x?=w190:bool)
      n53 = Initialize Array(0.0 ("offset"), w182) -> (w193:dbl[])
      n54 = Initialize Array(w185, w182) -> (w184:dbl[])
      n55 = Initialize Array(0.0 ("element"), w182) -> (w183:dbl[])
      n56 = Bundle By Name(cluster=T2 {"int32"=[], "int16"=[], "offset [smpl]"=0, "count [smpl]"=0, "is int16?"=FALSE, "all done?"=FALSE, "sampling?"=FALSE, "instr buffer [%]"=0.0, "queue buffer [%]"=0.0, "valid?"=FALSE} ("data"), "int32"=w187, "int16"=i16[][] [], "offset [smpl]"=w192, "count [smpl]"=w191, "is int16?"=FALSE, "all done?"=w179, "sampling?"=w190, "instr buffer [%]"=w199, "queue buffer [%]"=w199, "valid?"=TRUE) -> (w202:T2)
      n57 = Bundle By Name(cluster=T1 {"offset [V]"=[], "gain [V]"=[], "time stamp [s]"=[], "increment [s]"=0.0, "T smpl"=[], "T [deg C]"=[], "valid?"=FALSE, "abs timestamp"=timestamp(0 s since 1904-01-01)} ("aux data"), "offset [V]"=w193, "gain [V]"=w184, "time stamp [s]"=w183, "increment [s]"=w180, "T smpl"=i32[] [], "T [deg C]"=dbl[][] [], "valid?"=w179, "abs timestamp"=w178) -> (w197:T1)
    }
    frame Default {
    }
  }
  "error out" <- w7
  "adc session out" <- w8
  "fetching done?" <- w6
  "data packet" <- w5
  "aux data" <- w4
